vi "Run.vi"(8 "error in (no error)":errorcluster, 9 "Time Ratio used":dbl, 10 "Maze (0: Empty, -1: Enemy. >0: Teammate":i32[][](array[numeric]), 11 "TeamEffort in":refnum<class "TeamEffort.lvclass">) -> (0 "error out":errorcluster, 1 "Direction":T1, 2 "Action":T2, 3 "TeamEffort out":refnum<class "TeamEffort.lvclass">, 4 "Replicated":refnum<class "Square.lvclass">)   [LabVIEW 2015, in "TeamEffort.lvclass"]
uses:
  TeamEffort.lvclass
  Type Defs/Action Enum.ctl
  Type Defs/Direction Enum.ctl
  Square/Square.lvclass
  TeamEffort.lvclass/TeamEffort.ctl
  Type Defs/SB Type Defs.lvlib
panel:
  # "NOTICE - YOU MUST NOT REMOVE THIS NOTICE. PER THE FOLLOWING LICENSE, YOU MAY REPRODUCE THIS SOFTWARE PROVIDED YOU FOLLOW THE TERMS\nOF THE LICENSE.\n\n---BEGIN BSD LICENSE (http://opensource.org/licenses/BSD-2-Clause)---\nCopyright (c) 2015, Endigit, Inc. <robert@endigit.com>\nAll rights reserved.\n\nRedistribution and use in source and binary forms, with or without modification, are permitted provided that the following conditions are met:\n\n1. Redistributions of source code must retain the above copyright notice, this list of conditions and the following disclaimer.\n\n2. Redistributions in binary form must reproduce the above copyright notice, this list of conditions and the following disclaimer in the documentation and/or other \nmaterials provided with the distribution.\n\nTHIS SOFTWARE IS PROVIDED BY THE COPYRIGHT HOLDERS AND CONTRIBUTORS \"AS IS\" AND ANY EXPRESS OR IMPLIED WARRANTIES, INCLUDING, BUT NOT \nLIMITED TO, THE IMPLIED WARRANTIES OF MERCHANTABILITY AND FITNESS FOR A PARTICULAR PURPOSE ARE DISCLAIMED. IN NO EVENT SHALL THE COPYRIGHT \nHOLDER OR CONTRIBUTORS BE LIABLE FOR ANY DIRECT, INDIRECT, INCIDENTAL, SPECIAL, EXEMPLARY, OR CONSEQUENTIAL DAMAGES (INCLUDING, BUT NOT \nLIMITED TO, PROCUREMENT OF SUBSTITUTE GOODS OR SERVICES; LOSS OF USE, DATA, OR PROFITS; OR BUSINESS INTERRUPTION) HOWEVER CAUSED AND ON \nANY THEORY OF LIABILITY, WHETHER IN CONTRACT, STRICT LIABILITY, OR TORT (INCLUDING NEGLIGENCE OR OTHERWISE) ARISING IN ANY WAY OUT OF THE USE \nOF THIS SOFTWARE, EVEN IF ADVISED OF THE POSSIBILITY OF SUCH DAMAGE.\n---END BSD LICENSE---"
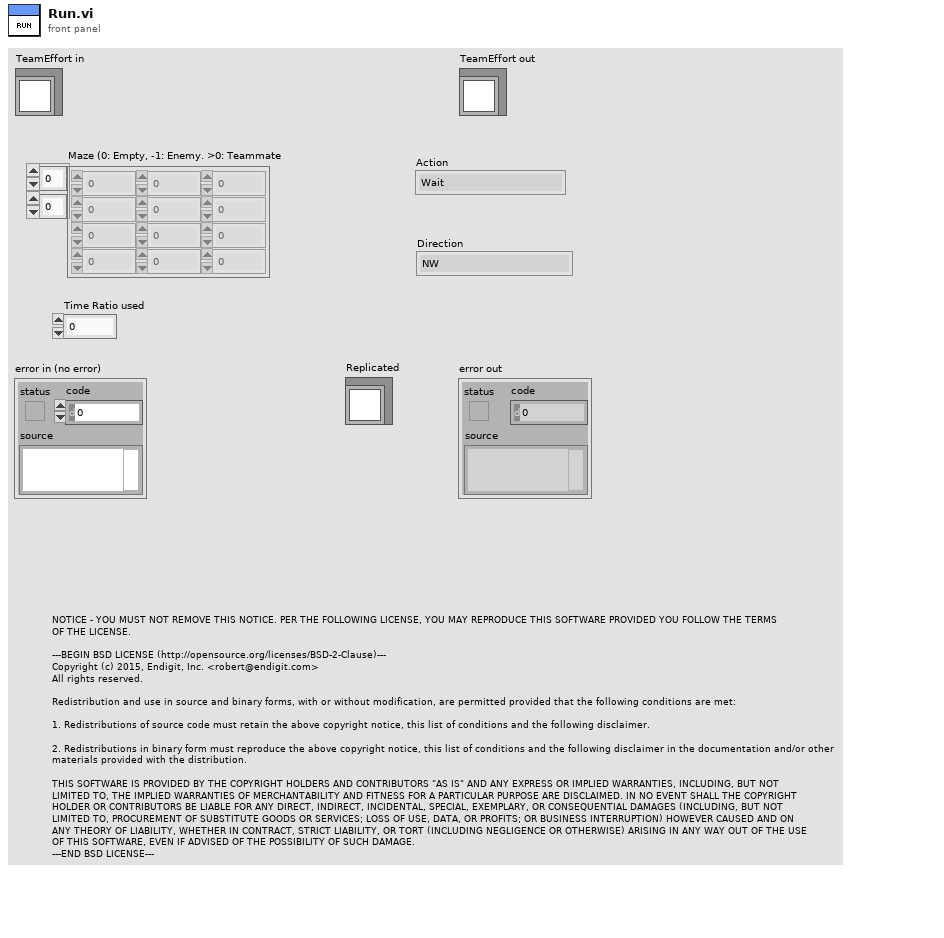
[diagram p1: front panel]
types:
  T1 = typedef "SB Type Defs.lvlib/Direction Enum.ctl" = enum16{"NW", "N", "NE", "E", "SE", "S", "SW", "W"}
  T2 = typedef "SB Type Defs.lvlib/Action Enum.ctl" = enum16{"Wait", "Move", "Attack", "Replicate"}
  T3 = typedef "TeamEffort.lvclass/Grid Cluster.ctl" = cluster{"p[x][y]":i32[][], "Move Count":i32, "Info[p]":T4[], "Known_p":i32}
  T4 = typedef "TeamEffort.lvclass/Player Cluster.ctl" = cluster{"Exp. Move":i32, "Moved?":bool, "In":T5, "Out":T6}
  T5 = typedef "TeamEffort.lvclass/Team Move Input.ctl" = cluster{"PlayerID":i32, "Y":i32, "X":i32, "Last Move":i32, "LastAction":T2}
  T6 = typedef "TeamEffort.lvclass/Team Move Output.ctl" = cluster{"Action":T2, "Direction":T1, "Replicated":refnum<class "Square.lvclass">}
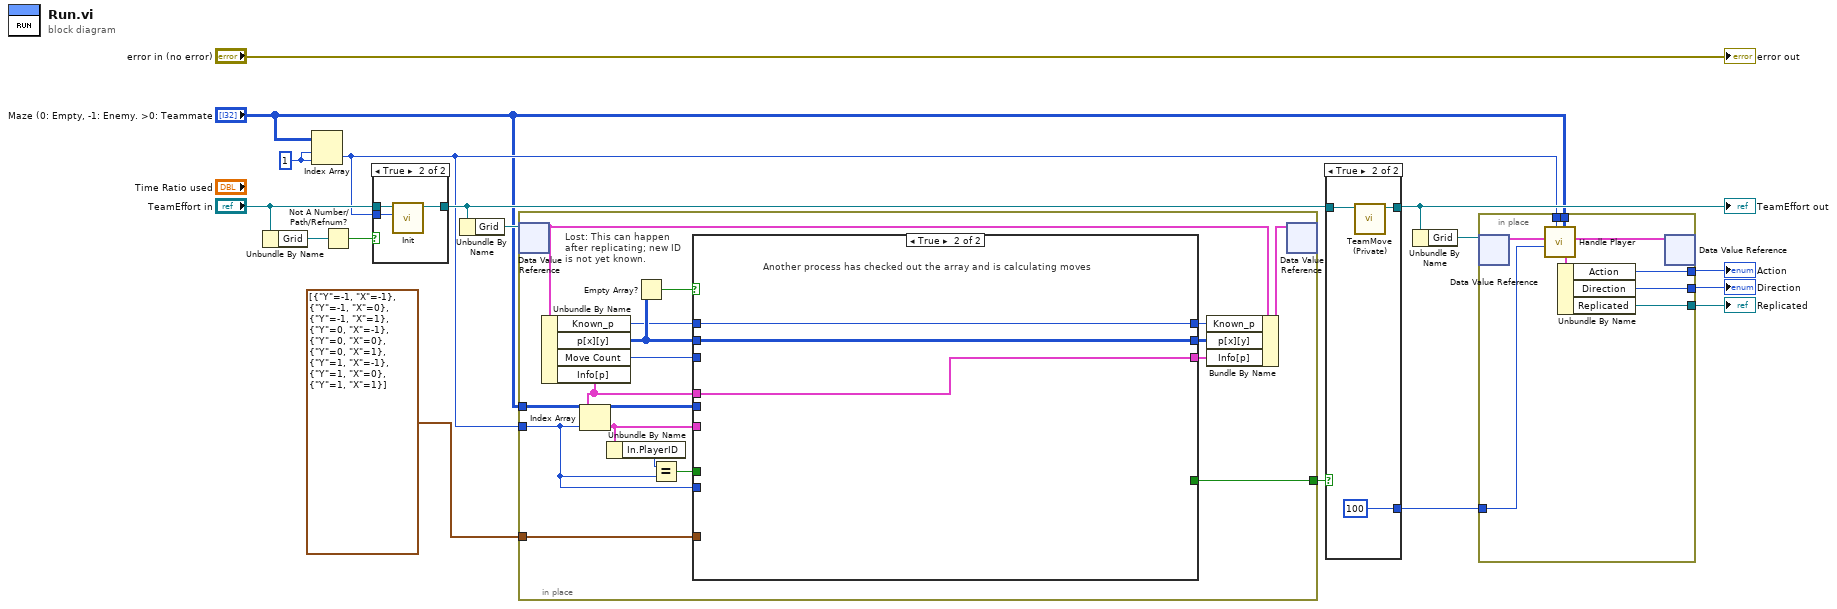
[diagram p0: block diagram]
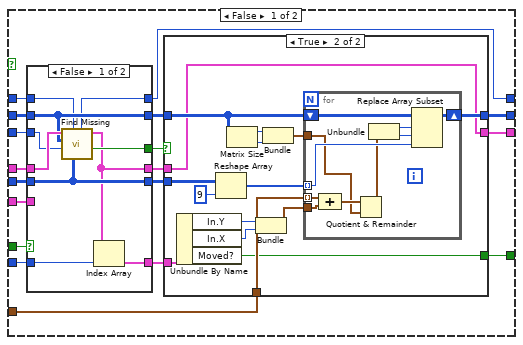
[diagram p4: hidden frame]
diagram:
  w14 = 1
  n1 = Unbundle By Name("TeamEffort in") -> ("Grid"=w17:refnum<data-value>)
  n2 = Index Array(array="Maze (0: Empty, -1: Enemy. >0: Teammate", index (row)=w14, index (col)=w14) -> (element=w2:i32)
  n3 = Not A Number/Path/Refnum?(number/path/refnum=w17) -> (NaN/Path/Refnum?=w11:bool)
  n4 = case shown="True" w11 {
    tunnel: "TeamEffort in" -> [w18 w21]
    tunnel: [w18 w20] -> w12
    tunnel: w2 -> [_ w19]
    frame False {
    }
    frame True {
      n5 = call-dynamic "Init.vi"("Player ID"=w19, "TeamEffort in"=w21) -> ("TeamEffort out"=w20:refnum<class "TeamEffort.lvclass">)  [unwired: 7 in, 2 out]
    }
  }
  n6 = Unbundle By Name(w12) -> ("Grid"=w15:refnum<data-value>)
  n7 = in-place {
    in-place-border: w2 -> [w27]
    in-place-border: [w26] -> w10
    in-place-border: "Maze (0: Empty, -1: Enemy. >0: Teammate" -> [w33]
    in-place-border: cluster{"Y":i32, "X":i32}[] [{"Y"=-1, "X"=-1}, {"Y"=-1, "X"=0}, {"Y"=-1, "X"=1}, {"Y"=0, "X"=-1}, {"Y"=0, "X"=0}, {"Y"=0, "X"=1}, {"Y"=1, "X"=-1}, {"Y"=1, "X"=0}, {"Y"=1, "X"=1}] -> [w36]
    # "Lost: This can happen after replicating; new ID is not yet known."
    n8 = in-place-dvr #1(w15) -> (w38:T3)  [unwired: 1 out]
    n9 = Unbundle By Name(w38) -> ("Known_p"=w22:i32, "p[x][y]"=w24:i32[][], "Move Count"=w30:i32, "Info[p]"=w31:T4[])
    n10 = Index Array(array=w31, index=w27) -> (element=w29:T4)
    n11 = Unbundle By Name(w29) -> ("In.PlayerID"=w34:i32)
    n12 = Empty Array?(array=w24) -> (empty?=w23:bool)
    n13 = Equal?(x=w34, y=w27) -> (x = y?=w32:bool)
    n14 = case shown="True" w23 {
      tunnel: w36 -> [w56 _]
      tunnel: [w55 w100] -> w35
      tunnel: w33 -> [w54 _]
      tunnel: w32 -> [w53 _]
      tunnel: w31 -> [w50 w101]
      tunnel: w30 -> [w49 _]
      tunnel: w29 -> [w48 _]
      tunnel: [w44 w101] -> w28
      tunnel: w27 -> [w43 _]
      tunnel: [w42 _] -> w26
      tunnel: w22 -> [w41 w102]
      tunnel: [w40 w102] -> w25
      tunnel: w24 -> [w39 w100]
      frame False {
        n15 = case shown="False" w53 {
          selector: w53 -> [_ w96]
          tunnel: [w89 w99] -> w45
          tunnel: w39 -> [w86 w98]
          tunnel: w50 -> [w93 w99]
          tunnel: w54 -> [w92 w97]
          tunnel: [w86 w98] -> w52
          tunnel: [w92 w97] -> w51
          tunnel: w49 -> [w91 _]
          tunnel: [w90 w96] -> w46
          tunnel: w48 -> [_ w95]
          tunnel: [w87 w95] -> w47
          tunnel: w43 -> [w88 _]
          tunnel: w41 -> [w85 w94]
          tunnel: [w84 w94] -> w40
          frame False {
            n16 = call "Find Missing.vi"("Maze (0: Empty, -1: Enemy. >0: Teammate"=w92, "known_p in"=w85, "Move"=w91, "Assumed Board"=w86, "Info[p]"=w93) -> ("Found?"=w90:bool, "Info[p] out"=w89:T4[], "known_p out"=w84:i32)  [unwired: 4 in]
            n17 = Index Array(array=w89, index=w88) -> (element=w87:T4)
          }
          frame True {
          }
        }
        n18 = case shown="True" w46 {
          tunnel: w56 -> [_ w73]
          tunnel: [w58 w72] -> w55
          tunnel: w52 -> [w58 w65]
          tunnel: w51 -> [_ w64]
          tunnel: [_ w61] -> w42
          tunnel: w47 -> [_ w60]
          tunnel: w45 -> [w57 w59]
          tunnel: [w57 w59] -> w44
          frame False {
          }
          frame True {
            n19 = Unbundle By Name(w60) -> ("In.Y"=w63:i32, "In.X"=w62:i32, "Moved?"=w61:bool)
            n20 = Reshape Array(w64, 9 ("dimension size")) -> (w66:i32[])
            n21 = Matrix Size(0:w65) -> (1:w70:i32, 2:w69:i32)
            n22 = Bundle("Y"=w63, "X"=w62) -> (w71:cluster{"Y":i32, "X":i32})  [unwired: 1 in]
            n23 = Bundle("number of columns"=w70, "matrix"=w69) -> (w68:cluster{"number of columns":i32, "matrix":i32})  [unwired: 1 in]
            n24 = for {
              shift-right: [w82] -> w72
              shift-left: w65 -> [w83]
              tunnel: w73 -> [w81] mode=indexing
              tunnel: w66 -> [w79] mode=indexing
              tunnel: w71 -> [w80]
              tunnel: w68 -> [w77]
              n25 = Compound Arithmetic op=ADD(w81, w80) -> (w78:cluster{"Y":i32, "X":i32})
              n26 = Quotient & Remainder(x=w78, y=w77) -> (x-y*floor(x/y)=w76:cluster{i32, i32})  [unwired: 1 out]
              n27 = Unbundle(w76) -> (w75:i32, w74:i32)
              n28 = Replace Array Subset(array=w83, new element=w79, index (row)=w75, index (col)=w74) -> (w82:i32[][])
            }
          }
        }
      }
      frame True {
        # "Another process has checked out the array and is calculating moves"
      }
    }
    n29 = Bundle By Name(cluster=w38, "Known_p"=w25, "p[x][y]"=w35, "Info[p]"=w28) -> (w37:T3)
    n30 = in-place-dvr #1(w37) -> ()  [unwired: 2 out]
  }
  n31 = case shown="True" w10 {
    tunnel: [w103 w106] -> w9
    tunnel: w12 -> [w103 w105]
    tunnel: [_ 100] -> w3
    frame False {
    }
    frame True {
      n32 = call "TeamMove (Private).vi"("TeamEffort in"=w105) -> ("TeamEffort out"=w106:refnum<class "TeamEffort.lvclass">)  [unwired: 9 in, 1 out]
    }
  }
  "TeamEffort out" <- w9
  n33 = Unbundle By Name(w9) -> ("Grid"=w8:refnum<data-value>)
  n34 = in-place {
    in-place-border: [w108] -> w6
    in-place-border: [w109] -> w5
    in-place-border: [w110] -> w4
    in-place-border: w3 -> [w112]
    in-place-border: w2 -> [w113]
    in-place-border: "Maze (0: Empty, -1: Enemy. >0: Teammate" -> [w107]
    n35 = in-place-dvr #2(w8) -> (w115:T3)  [unwired: 1 out]
    n36 = call "Handle Player.vi"("Maze (0: Empty, -1: Enemy. >0: Teammate"=w107, "p"=w113, "Additional Wait"=w112, "Data"=w115) -> ("Output"=w111:T6, "Data out"=w114:T3)  [unwired: 6 in]
    n37 = Unbundle By Name(w111) -> ("Action"=w108:T2, "Direction"=w109:T1, "Replicated"=w110:refnum<class "Square.lvclass">)
    n38 = in-place-dvr #2(w114) -> ()  [unwired: 2 out]
  }
  "Action" <- w6
  "Direction" <- w5
  "Replicated" <- w4
  "error out" <- "error in (no error)"
